vi "Test Get Summary of Case.vi"(8 "error in (no error)":errorcluster, 11 "Result Model Result Recording Test in":refnum<class "Result Model Result Recording Test.lvclass">) -> (0 "error out":errorcluster, 3 "Result Model Result Recording Test out":refnum<class "Result Model Result Recording Test.lvclass">)   [LabVIEW 2020, in "Result Model Result Recording Test.lvclass"]
uses:
  Result Model Result Recording Test.lvclass
  Result Model Result Recording Test.lvclass/Result Model Result Recording Test.ctl
  source/Core/Result/Type.ctl
  source/Core/Result/Result.lvlib
  source/Core/Result/Status.ctl
  source/Core/Result/Result.ctl
  ae2c71b8-32bb-49d1-8500-0119bfec74ff.vi
  source/User Interface/Result Model/Result Model.lvclass
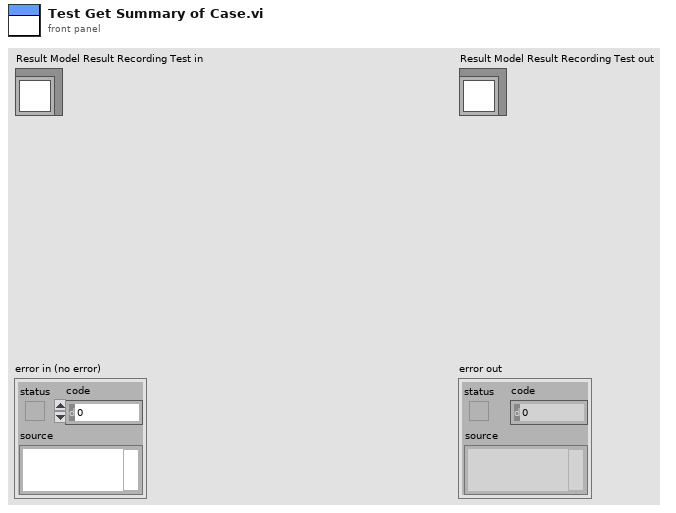
[diagram p1: front panel]
types:
  T1 = typedef "Result.lvlib/Result.ctl" = cluster{"Name":string, "Message":string, "Description":string, "Status":T2, "Result Type":T3, "Execution Time":dbl}
  T2 = typedef "Result.lvlib/Status.ctl" = enum16{"", "Passed", "Failed", "Error", "Skipped", "Setup Error", "Broken", "Teardown Error"}
  T3 = typedef "Result.lvlib/Type.ctl" = enum16{"Test Case", "Test Suite", "Test Run", "Pass", "Fail", "Skip", "Pass if", "Fail if", "Pass if Error", "Fail if Error", "Pass if Equal", "Fail if Equal"}
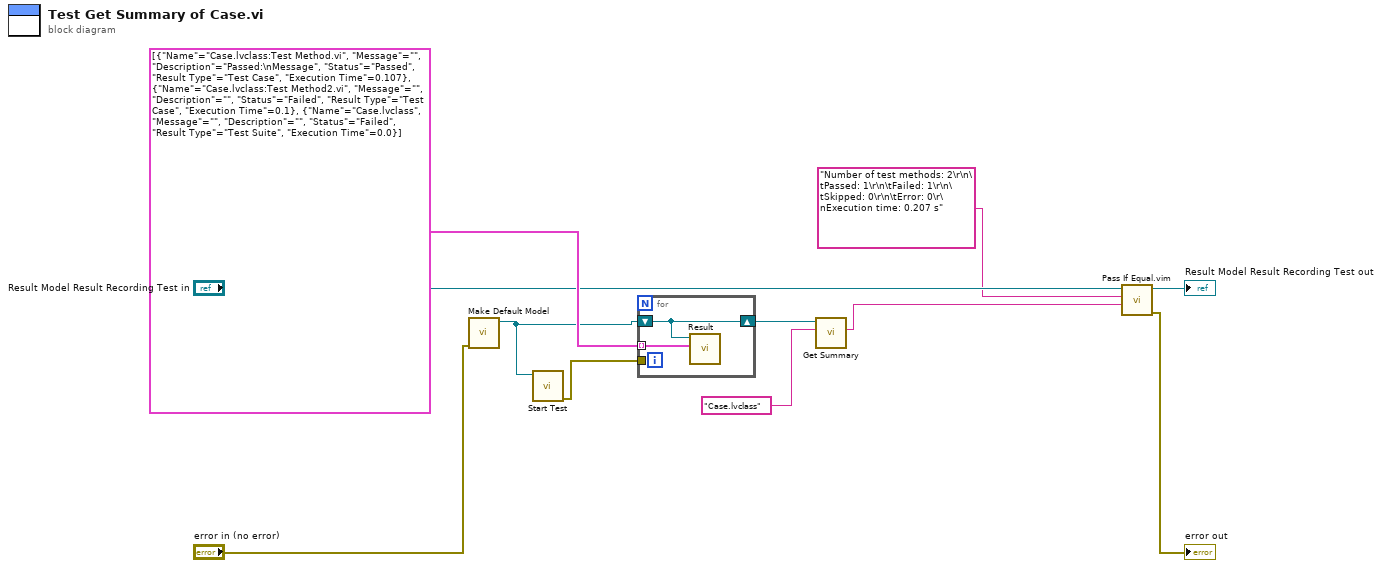
[diagram p0: block diagram]
diagram:
  n1 = call "Make Default Model.vi"("error in (no error)"="error in (no error)") -> ("Result Model out"=w2:refnum<class "Result Model.lvclass">)  [unwired: 9 in, 1 out]
  n2 = call "Start Test.vi"("Result Model In"=w2) -> ("error out"=w1:errorcluster)  [unwired: 10 in]
  n3 = for {
    tunnel: T1[] [{"Name"="Case.lvclass:Test Method.vi", "Message"="", "Description"="Passed:\nMessage", "Status"=enum."Passed", "Result Type"=enum."Test Case", "Execution Time"=0.107}, {"Name"="Case.lvclass:Test Method2.vi", "Message"="", "Description"="", "Status"=enum."Failed", "Result Type"=enum."Test Case", "Execution Time"=0.1}, {"Name"="Case.lvclass", "Message"="", "Description"="", "Status"=enum."Failed", "Result Type"=enum."Test Suite", "Execution Time"=0.0}] ("Results") -> [w13] mode=indexing
    shift-right: [w12] -> w5
    shift-left: w2 -> [w12]
    tunnel: w1 -> [_]
    n4 = call-dynamic "Result.vi"("Results"=w13, "Result Model in"=w12) -> ()  [unwired: 9 in, 1 out]
  }
  n5 = call "Get Summary.vi"("Item"="Case.lvclass", "Result Model In"=w5) -> ("Summary"=w3:string)  [unwired: 8 in, 1 out]
  n6 = call "Pass If Equal.vim"("Actual"=w3, "Expected"="Number of test methods: 2\r\n\tPassed: 1\r\n\tFailed: 1\r\n\tSkipped: 0\r\n\tError: 0\r\nExecution time: 0.207 s", "LUnit Test Case In"="Result Model Result Recording Test in") -> ("error out"=→"error out":errorcluster, "LUnit Test Case Out"=→"Result Model Result Recording Test out":refnum<class "Result Model Result Recording Test.lvclass">)  [unwired: 7 in]
